vi "sub_SparePinCheck.vi"(7 "ROI":T2, 8 "에러 입력(에러 없음)":errorcluster, 9 "추가된 배열":T1[](array[typedef]), 10 "BCG Values":T3={"Brightness"=171.0, "Contrast"=56.0, "Gamma"=2.0} {"Gamma" min=0.1 max=10 step=0.01 scale=10.0..0.1; "Contrast" min=1 max=89 step=1 scale=30.0..60.0; "Brightness" min=0 max=255 step=1 scale=0.0..255.0}, 11 "Image Src":T1) -> (0 "error out":errorcluster, 1 "최대값":u32, 2 "불리언":bool, 3 "Histogram":u32[](array[numeric]), 5 "Image Dst Out":T1)   [LabVIEW 2014]
uses:
  <vilib>/vision/Image Controls.llb/IMAQ Image.ctl
  <vilib>/vision/NI_Vision_Development_Module.lvlib
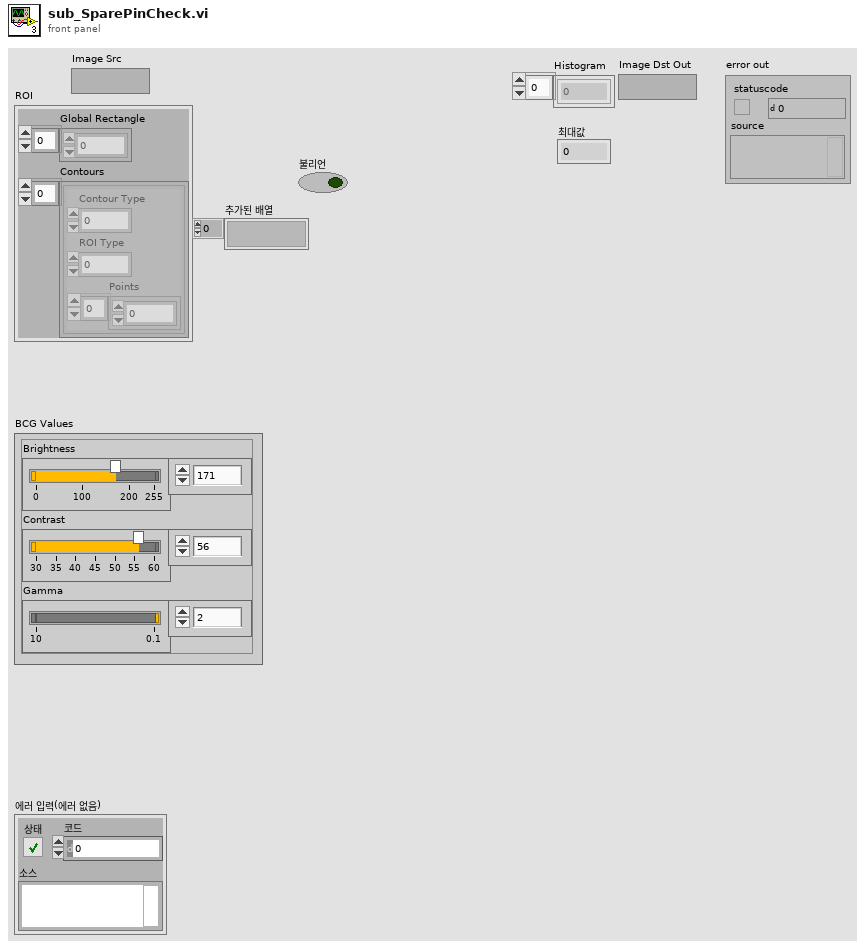
[diagram p1: front panel]
types:
  T1 = typedef "IMAQ Image.ctl" = refnum<image>
  T2 = cluster{"Global Rectangle":i32[], "Contours":cluster{"Contour Type":u32, "ROI Type":u32, "Points":i32[]}[]}
  T3 = cluster{"Brightness":sgl, "Contrast":sgl, "Gamma":sgl}
  T4 = cluster{"Starting Value":sgl, "Incremental Value":sgl, "Histogram":u32[]}
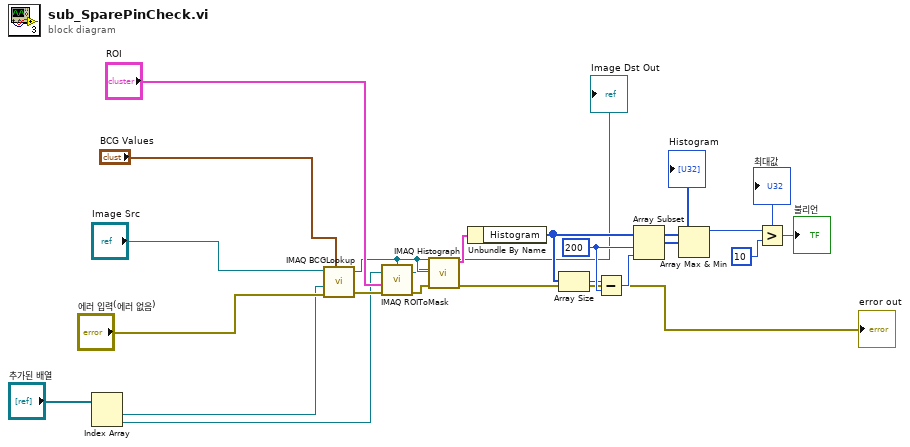
[diagram p0: block diagram]
diagram:
  w16 = 200 ("인덱스")
  n1 = Index Array(array="추가된 배열") -> (element #1=w4:T1, element #2=w3:T1)  [unwired: 2 in]
  n2 = call "IMAQ BCGLookup"("Image Src"="Image Src", "BCG Values"="BCG Values", "Image Dst"=w4, "error in (no error)"="에러 입력(에러 없음)") -> ("Image Dst Out"=w10:T1, "error out"=w11:errorcluster)  [unwired: 3 in]
  "Image Dst Out" <- w10
  n3 = call "IMAQ ROIToMask"("error in (no error)"=w11, "ROI Descriptor"="ROI", "Image"=w3, "Image Model"=w10) -> ("error out"=w8:errorcluster, "Image Out"=w9:T1)  [unwired: 2 in, 1 out]
  n4 = call "IMAQ Histograph"("error in (no error)"=w8, "Image Mask"=w9, "Image"=w10) -> ("error out"=→"error out":errorcluster, "Histogram Graph"=w13:T4)  [unwired: 5 in, 2 out]
  n5 = Unbundle By Name(w13) -> ("Histogram"=w14:u32[])
  "Histogram" <- w14
  n6 = Array Size(array=w14) -> (size(s)=w15:i32)
  n7 = Subtract(x=w15, y=w16) -> (x-y=w17:i32)
  n8 = Array Subset(array=w14, index=w16, length=w17) -> (w18:u32[])
  n9 = Array Max & Min(array=w18) -> (max value=w19:u32)  [unwired: 3 out]
  "최대값" <- w19
  n10 = Greater?(x=w19, y=u32 10) -> (0:→"불리언":bool)
